vi "Search Last Occurrence.vi"(9 "offset (0)":i32, 10 "search string/char (-)":string="-", 11 "string":string) -> (0 "offset of match":i32, 1 "rest of string":string, 2 "substring before match + match":string, 3 "substring before match":string)   [LabVIEW 2014, in "NIPM_API.lvlib"]
uses:
  NIPM_API.lvlib
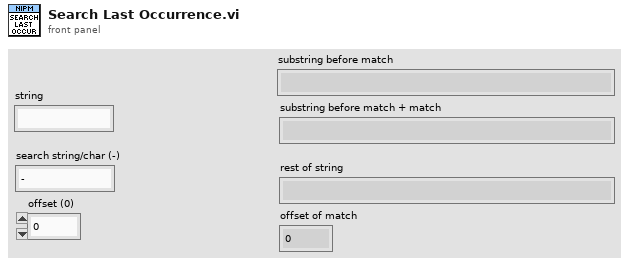
[diagram p1: front panel]
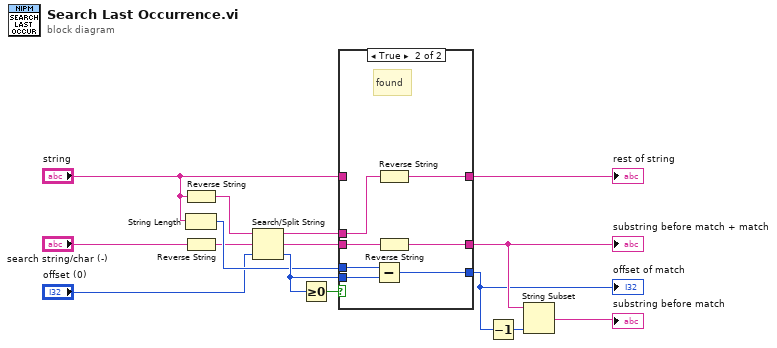
[diagram p0: block diagram]
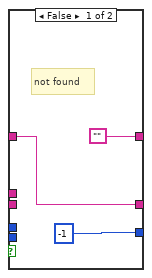
[diagram p2: hidden frame]
diagram:
  n1 = Reverse String(1:"string") -> (0:w7:string)
  n2 = String Length(string="string") -> (length=w9:i32)
  n3 = Reverse String(1:"search string/char (-)") -> (0:w8:string)
  n4 = Search/Split String(string=w7, search string/char (-)=w8, offset (0)="offset (0)") -> (substring before match=w14:string, match + rest of string=w15:string, offset of match=w12:i32)
  n5 = Greater Or Equal To 0?(x=w12) -> (x >= 0?=w10:bool)
  n6 = case shown="True" w10 {
    tunnel: w9 -> [_ w25]
    tunnel: "string" -> [w18 _]
    tunnel: [w18 w20] -> w4
    tunnel: w12 -> [_ w24]
    tunnel: [-1 w23] -> w2
    tunnel: ["" w19] -> w13
    tunnel: w14 -> [_ w22]
    tunnel: w15 -> [_ w21]
    frame False {
      # "not found"
    }
    frame True {
      # "found"
      n7 = Subtract(x=w25, y=w24) -> (x-y=w23:i32)
      n8 = Reverse String(1:w22) -> (0:w19:string)
      n9 = Reverse String(1:w21) -> (0:w20:string)
    }
  }
  "substring before match + match" <- w4
  "offset of match" <- w2
  "rest of string" <- w13
  n10 = Decrement(x=w2) -> (x-1=w1:i32)
  n11 = String Subset(string=w4, length (rest)=w1) -> (substring=→"substring before match":string)  [unwired: 1 in]
